vi "2.vi"   [LabVIEW 2020]
panel:
  # "2"
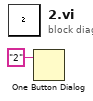
[diagram p0: block diagram]
diagram:
  n1 = One Button Dialog(message="2") -> ()  [unwired: 1 in, 1 out]
